vi "WriteIniFile.vi"(1 "value":string, 2 "key":string="FrontPanelPosition") -> ()   [LabVIEW 2014]
uses:
  <vilib>/Utility/config.llb/Write Key (String).vi
  <vilib>/Utility/config.llb/NI_LVConfig.lvlib
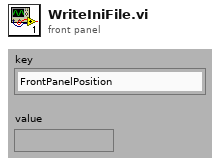
[diagram p1: front panel]
types:
  T1 = typedef "NI_LVConfig.lvlib/Config Data RefNum.ctl" = refnum<k1>
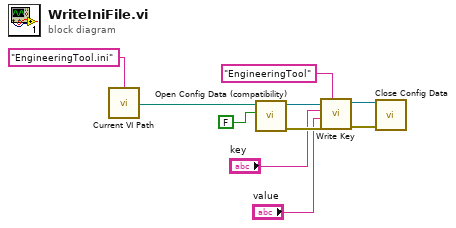
[diagram p0: block diagram]
diagram:
  n1 = call "Current VI Path.vi"("file name"="EngineeringTool.ini" ("name or relative path")) -> ("Path for file"=w1:path)
  n2 = call <vilib>:"Open Config Data (compatibility).vi"("create file if necessary (T)"=FALSE ("create file if necessary? (T)"), "configuration file path"=w1) -> ("error out"=w7:errorcluster, "refnum"=w10:T1)  [unwired: 7 in, 1 out]
  n3 = call-poly <vilib>:"Write Key.vi"("section"="EngineeringTool", "error in (no error)"=w7, "value"="value", "key"="key", "refnum"=w10) -> ("error out"=w5:errorcluster, "refnum out"=w6:T1)  [unwired: 4 in, 1 out]
  n4 = call <vilib>:"Close Config Data.vi"("error in (no error)"=w5, "refnum"=w6) -> ()  [unwired: 8 in, 2 out]
